vi "Camera.SaveImg.vi"(8 "error in (no error)":errorcluster, 10 "Path":path, 11 "Camera.Simulated":refnum<class "Camera.IMAQdx.lvclass">) -> (0 "error out":errorcluster, 3 "Camera.Simulated out":refnum<class "Camera.IMAQdx.lvclass">)   [LabVIEW 2020, in "Camera.IMAQdx.lvclass"]
doc: "---------------------------------------------------------------\nJKI State Machine Objects™\nhttp://jki.net/state-machine-objects/\nCopyright (C) 2005-2015, JKI <info@jki.net>\nALL RIGHTS RESERVEDJKI State Machine Objects (SMO) 1.0.0.5\nJKI - JKI\nCopyright (c) 2016, JKI"
uses:
  Camera.IMAQdx.lvclass
  <userlib>/_OpenG.lib/file/file.llb/Strip Path Extension - Path__ogtk.vi
  <vilib>/vision/driver/NI_Vision_Acquisition_Software.lvlib
  <vilib>/vision/driver/IMAQdx.llb/IMAQdx Buffer Number Mode.ctl
  Camera/Camera.lvclass
panel:
  # "For instructions on how to use the JKI State Machine Objects, examples and video tutorials, visit:\nhttp://jki.net/state-machine-objects/\n\nJKI State Machine Objects™\nhttp://jki.net/state-machine-objects/\nCopyright (C) 2005-2015, JKI <info@jki.net>\nALL RIGHTS RESERVED"
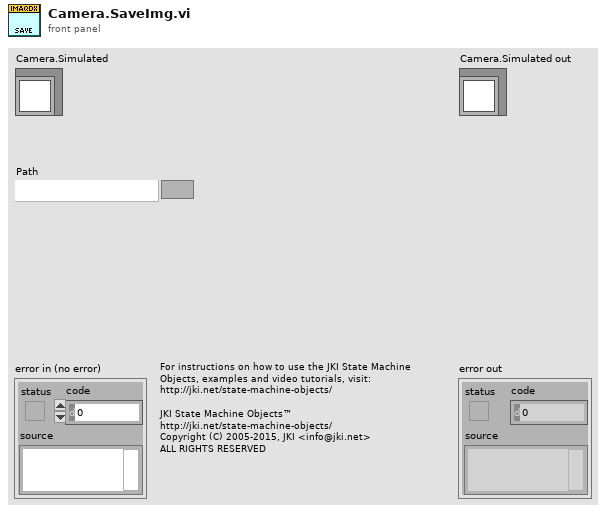
[diagram p1: front panel]
types:
  T1 = typedef "NI_Vision_Acquisition_Software.lvlib/IMAQdx Buffer Number Mode.ctl" = enum32{"Next", "Last", "Buffer Number", "Every", "Last New"}
  T2 = typedef "IMAQ Image.ctl" = refnum<image>
  T3 = typedef "IMAQdx.ctl" = refnum<k21>
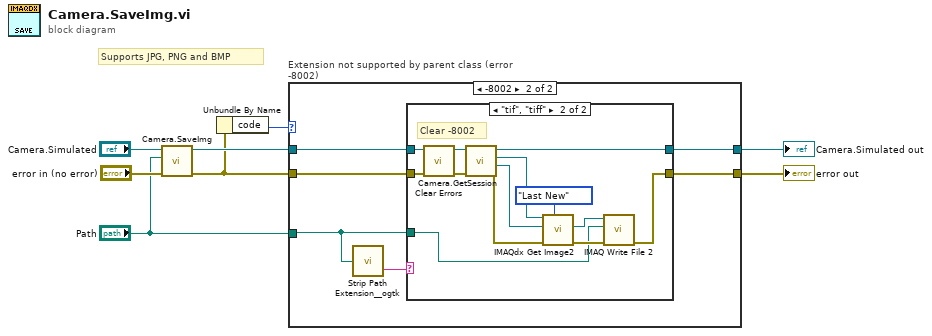
[diagram p0: block diagram]
diagram:
  # "Supports JPG, PNG and BMP"
  n1 = call-parent "Camera.SaveImg.vi"("error in (no error)"="error in (no error)", "Path"="Path", "Camera"="Camera.Simulated") -> ("error out"=w2:errorcluster, "Camera out"=w6:refnum<class "Camera.IMAQdx.lvclass">)  [unwired: 7 in]
  n2 = Unbundle By Name(w2) -> ("code"=w1:i32)
  n3 = case "Extension not supported by parent class (error -8002)" shown="-8002" w1 {
    tunnel: w2 -> [w9 w15]
    tunnel: w6 -> [w10 w16]
    tunnel: [w10 w12] -> w5
    tunnel: [w9 w13] -> w4
    tunnel: "Path" -> [_ w11]
    frame Default {
      # "File has been saved by parent implementation\nOr unexpected error."
    }
    frame -8002 {
      n4 = call-poly <userlib>:"Strip Path Extension__ogtk.vi"("path"=w11) -> ("extension"=w14:string)  [unwired: 1 out]
      n5 = case shown="\"tif\", \"tiff\"" w14 {
        tunnel: w16 -> [w18 w28]
        tunnel: w15 -> [w17 w30]
        tunnel: w11 -> [_ w22]
        tunnel: [w17 w20] -> w13
        tunnel: [w18 w19] -> w12
        frame Default {
          # "Don't clear the fault.\nThis VI does not support this extension"
        }
        frame "tif", "tiff" {
          # "Clear -8002"
          n6 = call <vilib>:"Clear Errors.vi"("error in (no error)"=w30) -> ("error out"=w24:errorcluster)  [unwired: 5 in, 1 out]
          n7 = call "Camera.GetSession.vi"("error in (no error)"=w24, "Camera.Simulated"=w28) -> ("error out"=w25:errorcluster, "Image"=w26:T2, "Session"=w27:T3, "Camera.Simulated"=w19:refnum<class "Camera.IMAQdx.lvclass">)  [unwired: 6 in]
          n8 = call <vilib>:"IMAQdx Get Image2.vi"("Buffer Number Mode (Next)"=IMAQdx_Buffer_Number_Mode."Last New", "error in"=w25, "Image In"=w26, "Session In"=w27) -> ("error out"=w23:errorcluster, "Image Out"=w21:T2)  [unwired: 4 in, 2 out]
          n9 = call-poly "IMAQ Write File 2"("error in (no error)"=w23, "File Path"=w22, "Image"=w21) -> ("error out"=w20:errorcluster)  [unwired: 7 in, 1 out]
        }
      }
    }
  }
  "error out" <- w4
  "Camera.Simulated out" <- w5
